vi "CleanUp.vi"(0 "object in":refnum<class "Database.lvclass">, 5 "error in (no error)":errorcluster) -> (14 "object out":refnum<class "Database.lvclass">, 19 "error out":errorcluster)   [LabVIEW 2015, in "Database.lvlib" / "Database.lvclass"]
uses:
  Database.lvclass
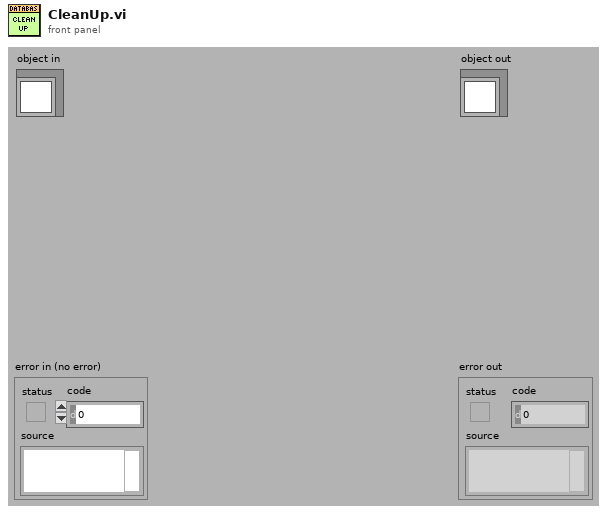
[diagram p1: front panel]
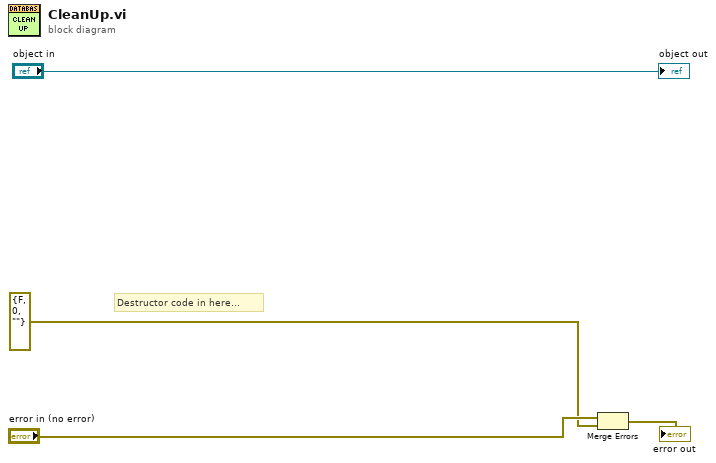
[diagram p0: block diagram]
diagram:
  # "Destructor code in here..."
  n1 = Merge Errors("error in (no error)", errorcluster {"status"=FALSE, "code"=0, "source"=""} ("error in (no error)")) -> (→"error out":errorcluster)
  "object out" <- "object in"
